vi "configuration_extended_audio.vi"() -> (3 "configuration_extended_audio":T1={"chunk"=512, "mixer_mode"=2, "loopback_gain"=1.0, "microphone_gain"=1.0, "profile"=3, "level"=41, "_reserved_0"=0, "_reserved_1"=0})   [LabVIEW 2023]
panel:
  in  "configuration_extended_audio":T1={"chunk"=512, "mixer_mode"=2, "loopback_gain"=1.0, "microphone_gain"=1.0, "profile"=3, "level"=41, "_reserved_0"=0, "_reserved_1"=0}
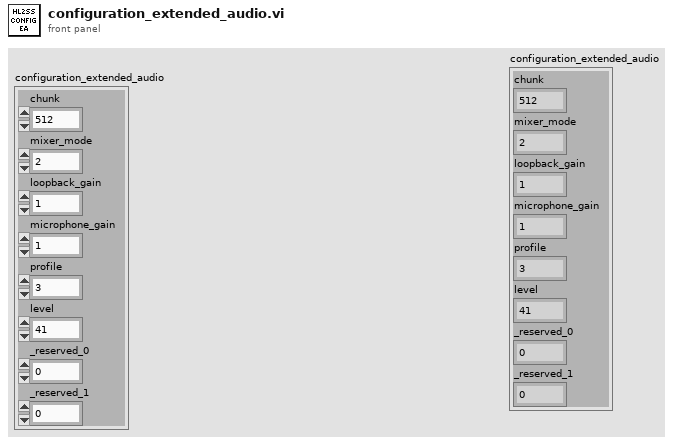
[diagram p1: front panel]
types:
  T1 = cluster{"chunk":u64, "mixer_mode":u32, "loopback_gain":sgl, "microphone_gain":sgl, "profile":u8, "level":u8, "_reserved_0":u8, "_reserved_1":u8}
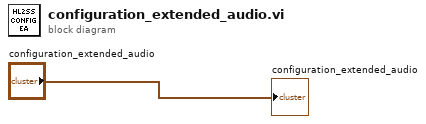
[diagram p0: block diagram]
diagram:
  "configuration_extended_audio" <- "configuration_extended_audio"
